vi "FrameClockGen.vi"(8 "Clock Period":u64) -> (0 "Pulse":bool, 4 "Pulse Start":bool)   [LabVIEW 2015]
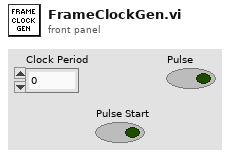
[diagram p1: front panel]
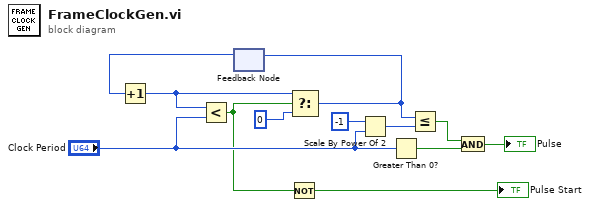
[diagram p0: block diagram]
diagram:
  n1 = feedback #1() -> (w3:u64)  [unwired: 1 in]
  n2 = Increment(x=w3) -> (x+1=w11:u64)
  n3 = Less?(x=w11, y="Clock Period") -> (x < y?=w2:bool)
  n4 = Not(x=w2) -> (.not. x?=→"Pulse Start":bool)
  n5 = Select(t=w11, s=w2, f=u64 0) -> (s? t:f=w4:u64)
  n6 = feedback-in #1(w4) -> ()
  n7 = Scale By Power Of 2(n=i16 -1, x="Clock Period") -> (x*2^n=w10:u64)
  n8 = Greater Than 0?(x="Clock Period") -> (x > 0?=w8:bool)
  n9 = Less Or Equal?(x=w4, y=w10) -> (x <= y?=w7:bool)
  n10 = And(x=w7, y=w8) -> (x .and. y?=→"Pulse":bool)
